vi "SetParameter.vi"(8 "error in (no error)":errorcluster, 10 "SetParameter":T1, 11 "ChromaPowerSupplyModel in":refnum<class "ChromaPowerSupplyModel.lvclass">) -> (0 "error out":errorcluster, 2 "StatusUpdates":string[](array[string]), 3 "ChromaPowerSupplyModel out":refnum<class "ChromaPowerSupplyModel.lvclass">)   [LabVIEW 2018, in "AcPwrPlugins.lvlib" / "ChromaPowerSupplyModel.lvclass"]
uses:
  ChromaPowerSupplyModel.lvclass
  AcPwrBaseClass/TypeDefs/SetParameterInputs.ctl
  AcPwrBaseClass/AcPwrBase.lvclass
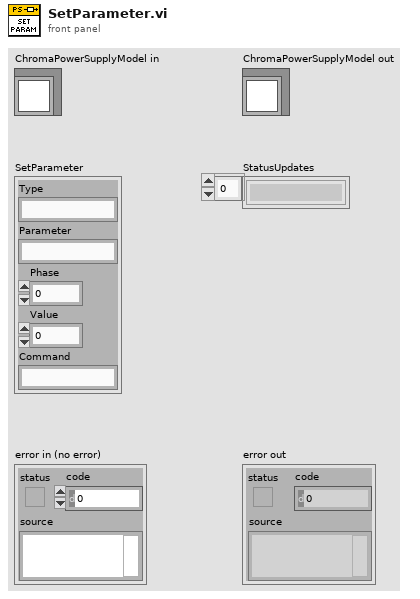
[diagram p1: front panel]
types:
  T1 = typedef "AcPwrPlugins.lvlib/AcPwrBase.lvclass/SetParameterInputs.ctl" = cluster{"Type":string, "Parameter":string, "Phase":i32, "Value":dbl, "Command":string}
  T2 = typedef "AcPwrPlugins.lvlib/ChromaPowerSupply.lvclass/Measurements.ctl" = cluster{"Handle":string, "Name":string, "Enabled":bool, "Measurement Value":dbl, "btnMeasFetch":bool, "ProtectionStatusString":string, "Measurement Type":enum16{"Voltage", "Current", "Power"}}[]
  T3 = typedef "AcPwrPlugins.lvlib/ChromaPowerSupply.lvclass/Device(s)Settings.ctl" = cluster{"Phases":cluster{"Handle":string, "Instrument Options":string, "id query (T)":bool, "reset device (T)":bool, "Timing":cluster{"TimingOn":enum16{""}, "Hours":u32, "Minutes":u32, "Seconds":dbl, "CutoffVoltage":dbl}, "Connected":bool, "Output Mode":enum16{"Voltage (DC)", "Current (DC)"}, "Voltage":dbl, "Current":dbl, "Voltage Limit":dbl, "Current Limit":dbl, "Power Protect":dbl, "Current Protect":dbl, "Voltage Protect":dbl}[], "MeasName":string}
  T4 = typedef "AcPwrPlugins.lvlib/ChromaPowerSupplyModel.lvclass/Database Settings.ctl" = cluster{"Data Source":string, "ICDAS to Model Table":string, "Model to ICDAS Table":string}
  T5 = cluster{"Handle":string, "Instrument Options":string, "id query (T)":bool, "reset device (T)":bool, "Timing":cluster{"TimingOn":enum16{""}, "Hours":u32, "Minutes":u32, "Seconds":dbl, "CutoffVoltage":dbl}, "Connected":bool, "Output Mode":enum16{"Voltage (DC)", "Current (DC)"}, "Voltage":dbl, "Current":dbl, "Voltage Limit":dbl, "Current Limit":dbl, "Power Protect":dbl, "Current Protect":dbl, "Voltage Protect":dbl}[]
  T6 = cluster{"Handle":string, "Instrument Options":string, "id query (T)":bool, "reset device (T)":bool, "Timing":cluster{"TimingOn":enum16{""}, "Hours":u32, "Minutes":u32, "Seconds":dbl, "CutoffVoltage":dbl}, "Connected":bool, "Output Mode":enum16{"Voltage (DC)", "Current (DC)"}, "Voltage":dbl, "Current":dbl, "Voltage Limit":dbl, "Current Limit":dbl, "Power Protect":dbl, "Current Protect":dbl, "Voltage Protect":dbl}
  T7 = cluster{"Device Settings":T3, "Database Settings":T4}
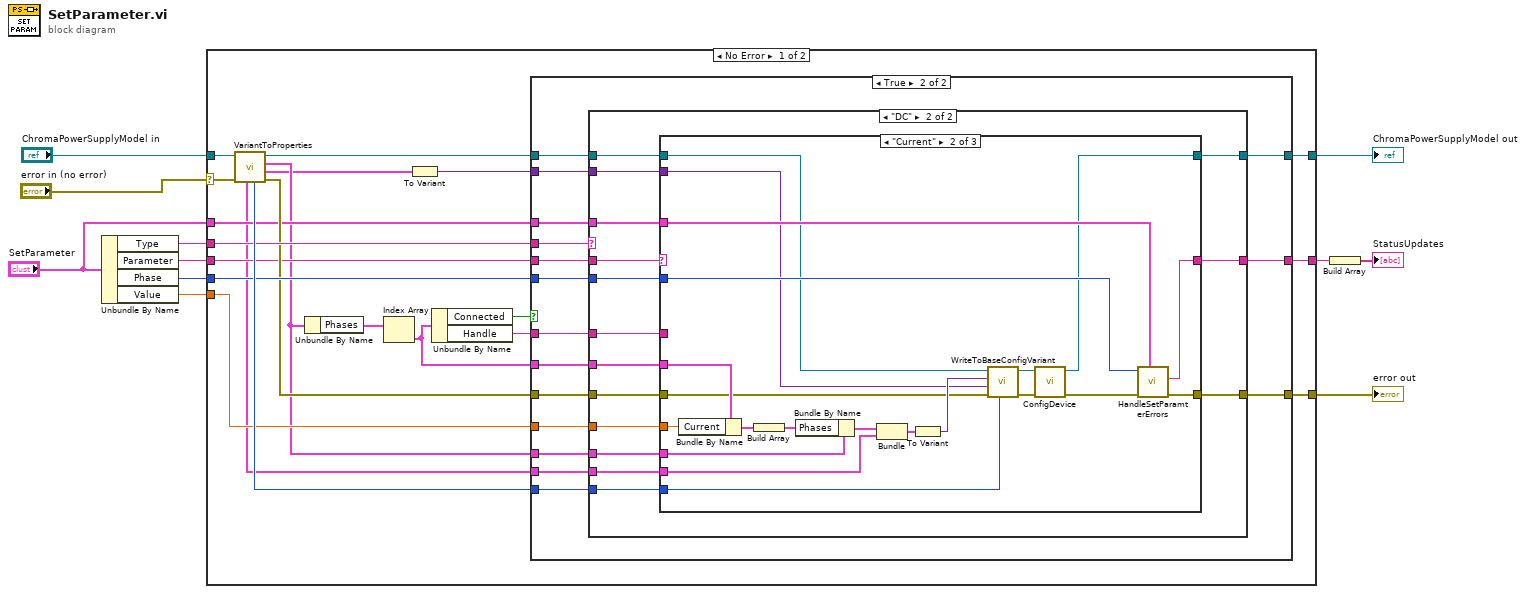
[diagram p0: block diagram]
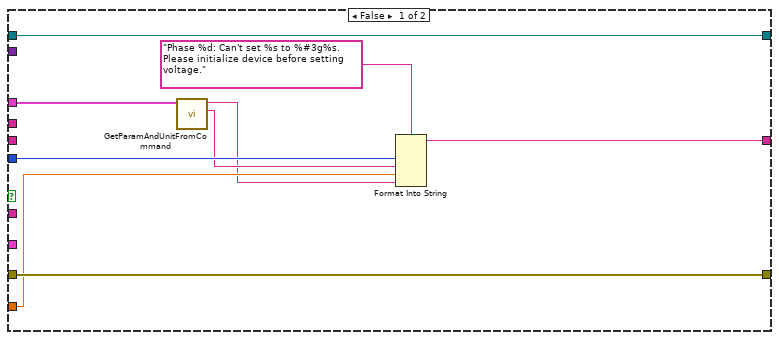
[diagram p2: hidden frame]
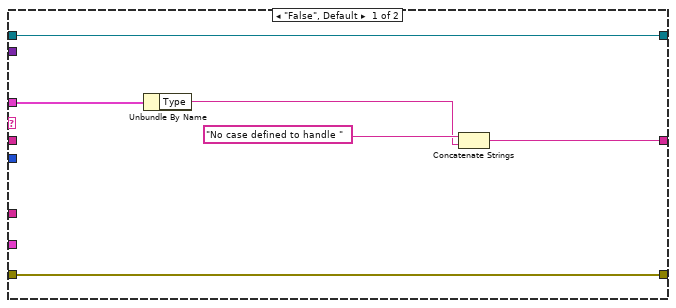
[diagram p3: hidden frame]
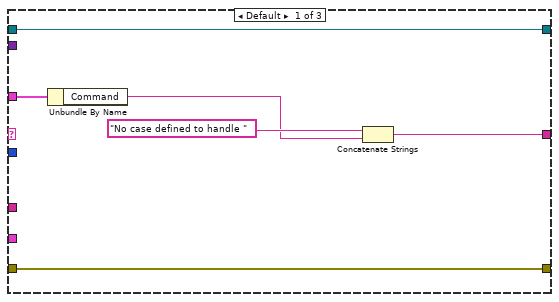
[diagram p4: hidden frame]
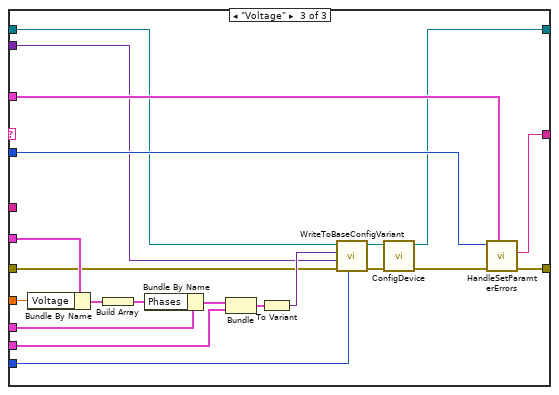
[diagram p5: hidden frame]
diagram:
  n1 = Unbundle By Name("SetParameter") -> ("Type"=w9:string, "Parameter"=w8:string, "Phase"=w11:i32, "Value"=w10:dbl)
  n2 = case shown="No Error" "error in (no error)" {
    selector: "error in (no error)" -> [w26 w128]
    tunnel: "ChromaPowerSupplyModel in" -> [w32 w127]
    tunnel: [w14 w127] -> w5
    tunnel: w11 -> [w29 _]
    tunnel: [w28 _] -> w4
    tunnel: w9 -> [w27 _]
    tunnel: [w24 w128] -> w3
    tunnel: w10 -> [w23 _]
    tunnel: w8 -> [w22 _]
    tunnel: "SetParameter" -> [w21 _]
    frame No Error {
      n3 = call "VariantToProperties.vi"("error in (no error)"=w26, "ChromaPowerSupplyModel in"=w32) -> ("error out"=w25:errorcluster, "Measurements"=w17:T2, "Device Settings"=w19:T3, "ChromaPowerSupplyModel out"=w15:refnum<class "ChromaPowerSupplyModel.lvclass">, "Measurement Refresh Time (ms)"=w30:u32, "Database Settings"=w18:T4)  [unwired: 4 in]
      n4 = Unbundle By Name(w19) -> ("Phases"=w20:T5)
      n5 = Index Array(array=w20) -> (element=w31:T6)  [unwired: 1 in]
      n6 = To Variant(anything=w17) -> (Variant=w16:variant)
      n7 = Unbundle By Name(w31) -> ("Connected"=w13:bool, "Handle"=w12:string)
      n8 = case shown="True" w13 {
        tunnel: w25 -> [w41 w57]
        tunnel: [w41 w56] -> w24
        tunnel: w12 -> [_ w55]
        tunnel: w23 -> [w35 w54]
        tunnel: w30 -> [_ w53]
        tunnel: w29 -> [w40 w52]
        tunnel: [w38 w51] -> w28
        tunnel: w27 -> [_ w50]
        tunnel: w22 -> [_ w49]
        tunnel: w21 -> [w37 w48]
        tunnel: w15 -> [w33 w47]
        tunnel: w31 -> [_ w46]
        tunnel: w19 -> [_ w45]
        tunnel: w18 -> [_ w44]
        tunnel: w16 -> [_ w43]
        tunnel: [w33 w42] -> w14
        frame False {
          n9 = call "GetParamAndUnitFromCommand.vi"("SetParameter"=w37) -> ("Parameter"=w36:string, "Unit Label"=w34:string)  [unwired: 9 in]
          n10 = Format Into String(format string="Phase %d: Can't set %s to %#3g%s. Please initialize device before setting voltage.", w40, w36, w35, w34) -> (resulting string=w38:string)  [unwired: 2 in, 1 out]
        }
        frame True {
          n11 = case shown="\"DC\"" w50 {
            tunnel: w57 -> [w59 w78]
            tunnel: [w59 w77] -> w56
            tunnel: w55 -> [_ w76]
            tunnel: w54 -> [_ w75]
            tunnel: w53 -> [_ w74]
            tunnel: w52 -> [_ w73]
            tunnel: [w60 w72] -> w51
            tunnel: w49 -> [_ w71]
            tunnel: w48 -> [w61 w70]
            tunnel: w47 -> [w58 w69]
            tunnel: w46 -> [_ w68]
            tunnel: w45 -> [_ w67]
            tunnel: w44 -> [_ w66]
            tunnel: w43 -> [_ w65]
            tunnel: [w58 w64] -> w42
            frame "False", Default {
              n12 = Unbundle By Name(w61) -> ("Type"=w62:string)
              n13 = Concatenate Strings("No case defined to handle " ("string"), w62) -> (w60:string)
            }
            frame "DC" {
              n14 = case shown="\"Current\"" w71 {
                tunnel: w78 -> [w84 w89 w110]
                tunnel: [w84 w92 w113] -> w77
                tunnel: w76 -> [_ _ _]
                tunnel: w75 -> [_ w100 w121]
                tunnel: w74 -> [_ w86 w107]
                tunnel: w73 -> [_ w105 w126]
                tunnel: [w83 w104 w125] -> w72
                tunnel: w70 -> [w81 w103 w124]
                tunnel: w69 -> [w79 w96 w117]
                tunnel: w68 -> [_ w101 w122]
                tunnel: w67 -> [_ w99 w120]
                tunnel: w66 -> [_ w93 w114]
                tunnel: w65 -> [_ w88 w109]
                tunnel: [w79 w85 w106] -> w64
                frame Default {
                  n15 = Unbundle By Name(w81) -> ("Command"=w80:string)
                  n16 = Concatenate Strings("No case defined to handle " ("string"), w80) -> (w83:string)
                }
                frame "Current" {
                  n17 = Bundle By Name(cluster=w101, "Current"=w100) -> (w98:T6)
                  n18 = Build Array(w98) -> (w97:T5)
                  n19 = Bundle By Name(cluster=w99, "Phases"=w97) -> (w94:T3)
                  n20 = Bundle("Device Settings"=w94, "Database Settings"=w93) -> (w95:T7)  [unwired: 1 in]
                  n21 = To Variant(anything=w95) -> (Variant=w91:variant)
                  n22 = call-dynamic "WriteToBaseConfigVariant.vi"("Measurement Refresh Time (ms)"=w86, "error in (no error)"=w89, "Meas"=w88, "Config"=w91, "ChromaPowerSupplyModel in"=w96) -> ("error out"=w90:errorcluster, "ChromaPowerSupplyModel out"=w87:refnum<class "ChromaPowerSupplyModel.lvclass">)  [unwired: 5 in]
                  n23 = call-dynamic "ConfigDevice.vi"("error in (no error)"=w90, "ChromaPowerSupplyModel in"=w87) -> ("error out"=w102:errorcluster, "ChromaPowerSupplyModel out"=w85:refnum<class "ChromaPowerSupplyModel.lvclass">)  [unwired: 8 in]
                  n24 = call "HandleSetParamterErrors.vi"("SetParameter"=w103, "error in (no error)"=w102, "Phase"=w105) -> ("error IO"=w92:errorcluster, "Status Update"=w104:string)  [unwired: 7 in]
                }
                frame "Voltage" {
                  n25 = Bundle By Name(cluster=w122, "Voltage"=w121) -> (w119:T6)
                  n26 = Build Array(w119) -> (w118:T5)
                  n27 = Bundle By Name(cluster=w120, "Phases"=w118) -> (w115:T3)
                  n28 = Bundle("Device Settings"=w115, "Database Settings"=w114) -> (w116:T7)  [unwired: 1 in]
                  n29 = To Variant(anything=w116) -> (Variant=w112:variant)
                  n30 = call-dynamic "WriteToBaseConfigVariant.vi"("Measurement Refresh Time (ms)"=w107, "error in (no error)"=w110, "Meas"=w109, "Config"=w112, "ChromaPowerSupplyModel in"=w117) -> ("error out"=w111:errorcluster, "ChromaPowerSupplyModel out"=w108:refnum<class "ChromaPowerSupplyModel.lvclass">)  [unwired: 5 in]
                  n31 = call-dynamic "ConfigDevice.vi"("error in (no error)"=w111, "ChromaPowerSupplyModel in"=w108) -> ("error out"=w123:errorcluster, "ChromaPowerSupplyModel out"=w106:refnum<class "ChromaPowerSupplyModel.lvclass">)  [unwired: 8 in]
                  n32 = call "HandleSetParamterErrors.vi"("SetParameter"=w124, "error in (no error)"=w123, "Phase"=w126) -> ("error IO"=w113:errorcluster, "Status Update"=w125:string)  [unwired: 7 in]
                }
              }
            }
          }
        }
      }
    }
    frame Error {
    }
  }
  "error out" <- w3
  "ChromaPowerSupplyModel out" <- w5
  n33 = Build Array(w4) -> (→"StatusUpdates":string[])
